vi "FCI_Lip_Outer_Width.vi"(0 "Image":T10(plugin-control), 1 "Calibrated Image":T10, 2 "Blob Center":cluster{"Center X":dbl, "Center Y":dbl}, 3 "Line Options ROI Ref":T8={"Number of Lines"=1, "Type"=enum."First Edge Rake", "Min. Score"=10.0, "Max. Score"=1000.0, "Orientation"=5.0, "Angle Range"=70.0, "Angle Tolerance"=1.0, "Step Size"=3, "Min. SNR (db)"=0.0, "Min. Points (%)"=25.0, "Hough Iterations"=5} {"Min. Points (%)" min=0.0 max=100.0; "Min. SNR (db)" min=0.0; "Max. Score" min=0.0 max=1024.0; "Min. Score" min=0.0 max=1024.0 step=1.0}, 4 "Edge Options ROI Ref":T6={"Edge Polarity"=0, "Kernel Size"=3, "Width"=3, "Minimum Edge Strength"=50.0, "Interpolation Type"=enum."Zero Order", "Data Processing Method"=enum."Average"} {"Edge Polarity" items=["All Edges", "Rising Edges", "Falling Edges"]; "Minimum Edge Strength" format="%.2f"; "Width" step=2; "Kernel Size" step=2}, 5 "error in (no error)":errorcluster, 6 "Search Direction ROI Ref":u32=3, 7 "Edge Options ROI 1":T6={"Edge Polarity"=0, "Kernel Size"=3, "Width"=3, "Minimum Edge Strength"=50.0, "Interpolation Type"=enum."Bilinear Fixed", "Data Processing Method"=enum."Average"} {"Edge Polarity" items=["All Edges", "Rising Edges", "Falling Edges"]; "Minimum Edge Strength" format="%.2f"; "Width" step=2; "Kernel Size" step=2}, 8 "Reference ROI":T11 {"Contours"."Type" items=["No Selection", "Point", "Line", "Rectangle", "Oval", "Polygon", "Freehand Region", "Annulus", "Unused2", "Unused3", "Broken Line", "Freehand Line", "Rotated Rectangle"]}, 9 "Measurement ROI":T11 {"Contours"."Type" items=["No Selection", "Point", "Line", "Rectangle", "Oval", "Polygon", "Freehand Region", "Annulus", "Unused2", "Unused3", "Broken Line", "Freehand Line", "Rotated Rectangle"]}, 10 "Search Direction ROI 1":u16(ring)=2 items=["Left To Right", "Right To Left", "Top To Bottom", "Bottom To Top"]) -> (13 "Overlay Arrow Lines":T1, 14 "Lip Outer Width Real World":sgl, 15 "Perpendicular Lines Lip Outer":T4(array[cluster])=[{{"X"=55.0, "Y"=48.0}, {"X"=263.0, "Y"=104.0}}, {{"X"=53.0, "Y"=53.0}, {"X"=262.0, "Y"=109.0}}, {{"X"=52.0, "Y"=58.0}, {"X"=261.0, "Y"=113.0}}, {{"X"=51.0, "Y"=62.0}, {"X"=259.0, "Y"=118.0}}, {{"X"=49.0, "Y"=67.0}, {"X"=258.0, "Y"=123.0}}, {{"X"=48.0, "Y"=72.0}, {"X"=257.0, "Y"=128.0}}, {{"X"=47.0, "Y"=77.0}, {"X"=255.0, "Y"=133.0}}, {{"X"=46.0, "Y"=82.0}, {"X"=254.0, "Y"=138.0}}, {{"X"=44.0, "Y"=87.0}, {"X"=253.0, "Y"=142.0}}, {{"X"=43.0, "Y"=91.0}, {"X"=252.0, "Y"=147.0}}, {{"X"=42.0, "Y"=96.0}, {"X"=250.0, "Y"=152.0}}] {"?"."Y" format="%.2f"; "?"."X" format="%.2f"; "?"."Y" format="%.2f"; "?"."X" format="%.2f"}, 19 "error IO":errorcluster)   [LabVIEW 2019, in "Algorithm.lvclass"]
uses:
  FrameworkOverrides/Algorithm.lvclass
  <vilib>/vision/NI_Vision_Development_Module.lvlib
  <vilib>/vision/Measure.llb/Edge Polarity.ctl
  <vilib>/vision/Measure.llb/Edge Options.ctl
  <vilib>/vision/Image Controls.llb/IMAQ Image.ctl
  <vilib>/vision/Measure.llb/Straight Edge Process.ctl
  <vilib>/vision/Measure.llb/Straight Edge Options.ctl
panel:
  out "Second Overlay Line":T2
  out "First Overlay Line":T3
  out "Rectangle 2":T5 {"Rotation" min=-90.0 max=90.0 step=1.0 format="%.2f"; "Left" scale=0.0..1024.0; "Right" scale=0.0..1024.0}
  out "Rectangle":T5 {"Rotation" min=-90.0 max=90.0 step=1.0 format="%.2f"; "Left" scale=0.0..1024.0; "Right" scale=0.0..1024.0}
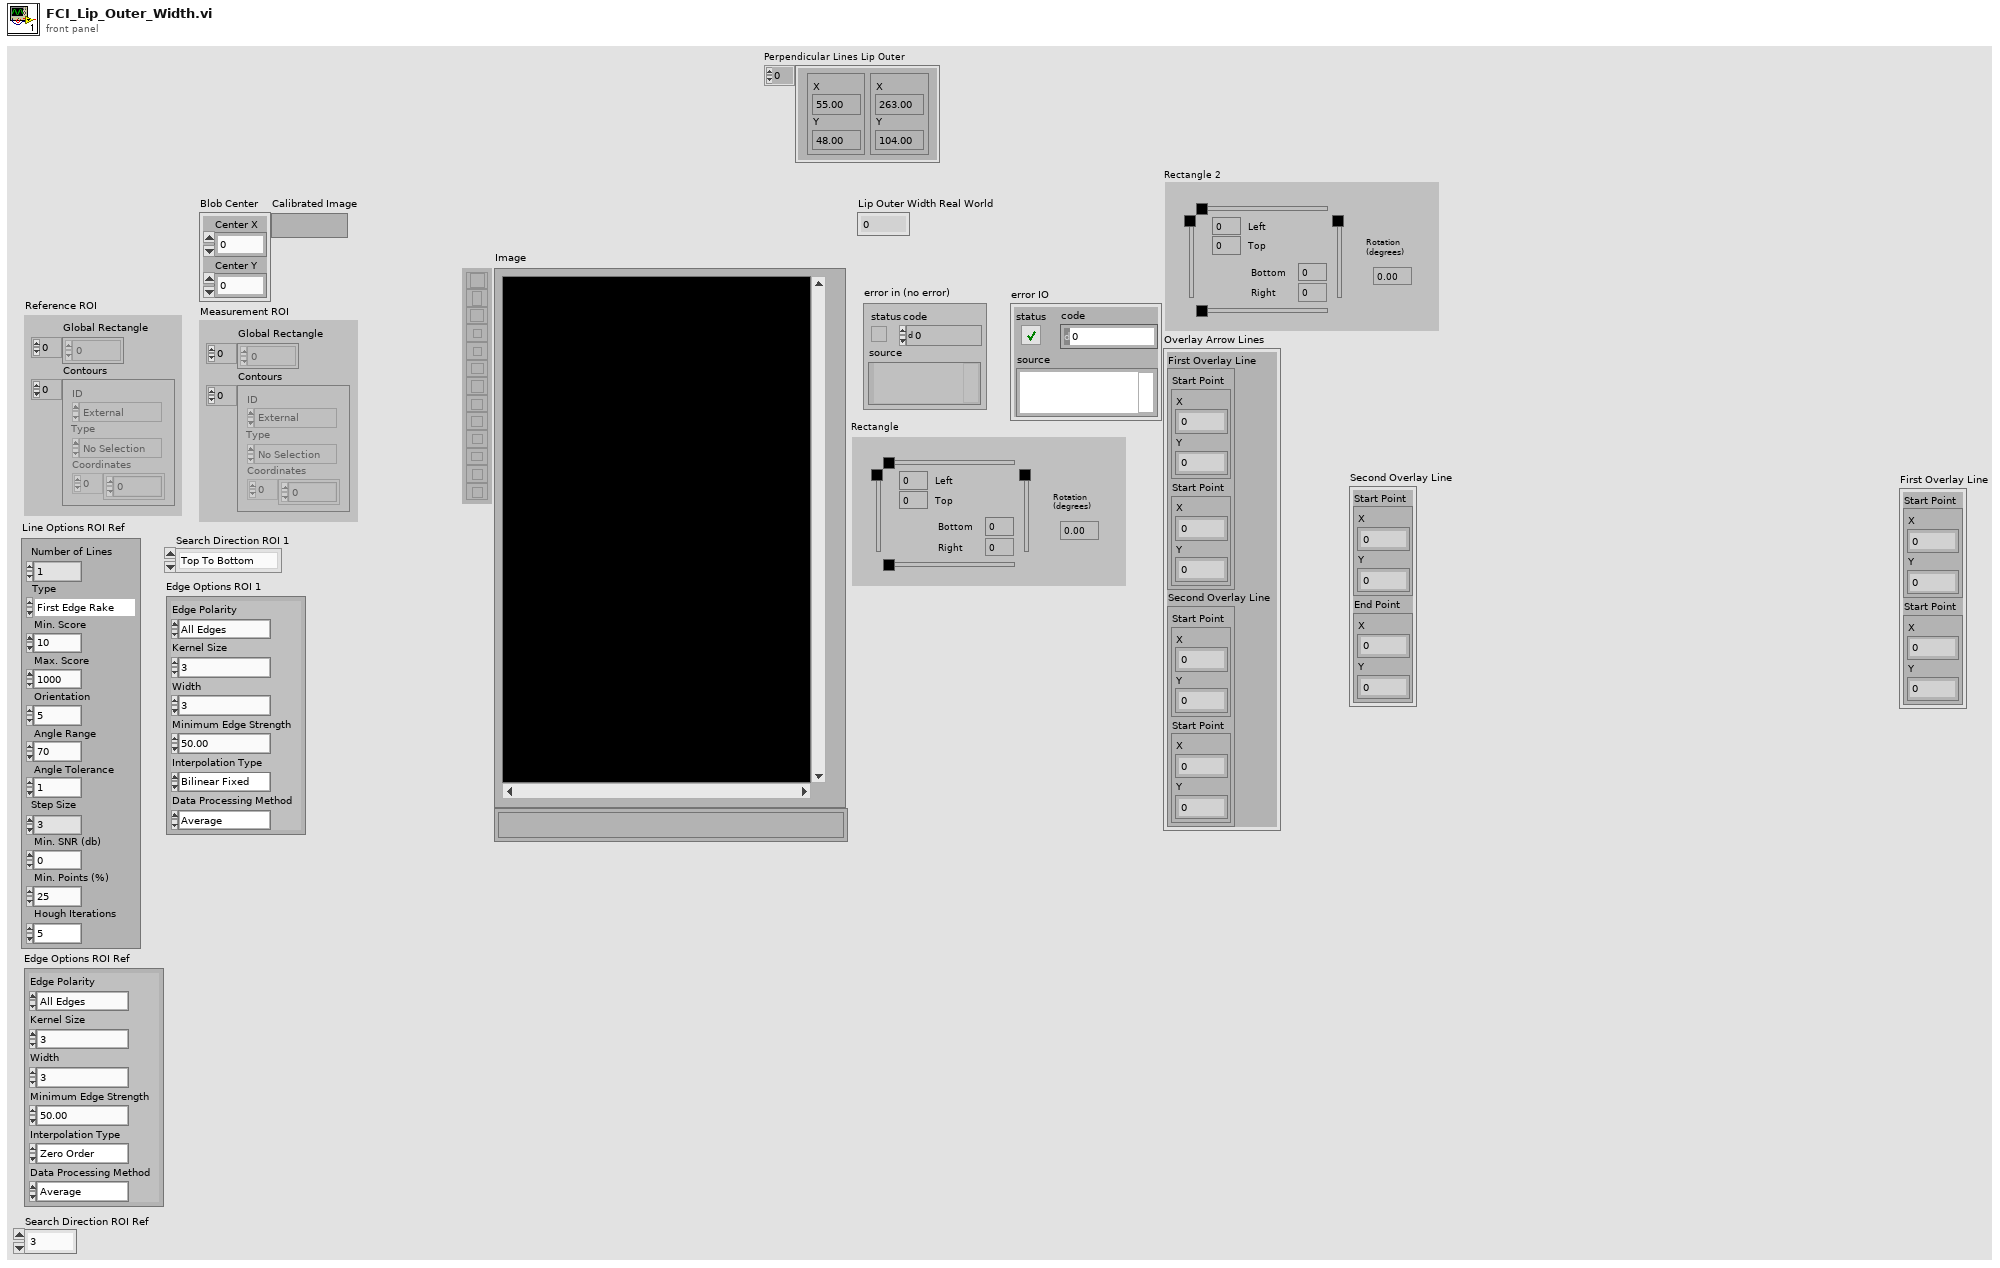
[diagram p1: front panel]
types:
  T1 = cluster{"First Overlay Line ":cluster{"Start Point":cluster{"X":sgl, "Y":sgl}, "Start Point":cluster{"X":sgl, "Y":sgl}}, "Second Overlay Line ":cluster{"Start Point":cluster{"X":sgl, "Y":sgl}, "Start Point":cluster{"X":sgl, "Y":sgl}}}
  T2 = cluster{"Start Point":cluster{"X":sgl, "Y":sgl}, "End Point":cluster{"X":sgl, "Y":sgl}}
  T3 = cluster{"Start Point":cluster{"X":sgl, "Y":sgl}, "Start Point":cluster{"X":sgl, "Y":sgl}}
  T4 = cluster{cluster{"X":sgl, "Y":sgl}, cluster{"X":sgl, "Y":sgl}}[]
  T5 = typedef "IMAQ Rectangle" = cluster{"Left":i32, "Top":i32, "Right":i32, "Bottom":i32, "Rotation":dbl}
  T6 = typedef "Edge Options.ctl" = cluster{"Edge Polarity":T7, "Kernel Size":u32, "Width":u32, "Minimum Edge Strength":sgl, "Interpolation Type":enum32{"Zero Order", "Bilinear", "Quadratic", "Cubic", "Bilinear Fixed"}, "Data Processing Method":enum32{"Average", "Median"}}
  T7 = typedef "Edge Polarity.ctl" = u32
  T8 = typedef "Straight Edge Options.ctl" = cluster{"Number of Lines":i32, "Type":T9, "Min. Score":dbl, "Max. Score":dbl, "Orientation":dbl, "Angle Range":dbl, "Angle Tolerance":dbl, "Step Size":u32, "Min. SNR (db)":dbl, "Min. Points (%)":dbl, "Hough Iterations":i32}
  T9 = typedef "Straight Edge Process.ctl" = enum32{"First Edge Rake", "Best Edge Rake", "Hough Edge Rake", "First Edge Projection", "Best Edge Projection"}
  T10 = typedef "IMAQ Image.ctl" = refnum<image>
  T11 = typedef "ROI Descriptor" = cluster{"Global Rectangle":i32[], "Contours":cluster{"ID":enum32{"External", "Internal"}, "Type":u32, "Coordinates":i32[]}[]}
  T12 = cluster{"Left":dbl, "Top":dbl, "Right":dbl, "Bottom":dbl, "Angle":dbl}
  T13 = cluster{"Search Direction":u32, "Edge Options":T6, "Show Search Area":bool, "Show Search Lines":bool, "Show Edges Found":bool, "Show Result":bool, "Search Area Color":u32, "Search Lines Color":u32, "Edge Locations Color":u32, "Result Color":u32, "Overlay Group Name":string}
  T14 = cluster{"Point1 (Pixels)":cluster{"X":sgl, "Y":sgl}, "Point2 (Pixels)":cluster{"X":sgl, "Y":sgl}, "Point1 (Real-World)":cluster{"X":sgl, "Y":sgl}, "Point2 (Real-World)":cluster{"X":sgl, "Y":sgl}, "Angle (Pixel)":dbl, "Angle (Real-World)":dbl, "Score":dbl, "Straightness":dbl, "Average SNR (db)":dbl, "Calibration Valid":bool}[]
  T15 = cluster{"Point1 (Pixels)":cluster{"X":sgl, "Y":sgl}, "Point2 (Pixels)":cluster{"X":sgl, "Y":sgl}, "Point1 (Real-World)":cluster{"X":sgl, "Y":sgl}, "Point2 (Real-World)":cluster{"X":sgl, "Y":sgl}, "Angle (Pixel)":dbl, "Angle (Real-World)":dbl, "Score":dbl, "Straightness":dbl, "Average SNR (db)":dbl, "Calibration Valid":bool}
  T16 = typedef "Search Line.ctl" = cluster{"Start Point":cluster{"X":sgl, "Y":sgl}, "End Point":cluster{"X":sgl, "Y":sgl}, "Edge Info":T17[], "Edge Map":dbl[], "Calibration Valid":bool}
  T17 = typedef "Edge New.ctl" = cluster{"Location (Pixel)":cluster{"X":sgl, "Y":sgl}, "Location (Real-World)":cluster{"X":sgl, "Y":sgl}, "Distance (Pixel)":dbl, "Distance (Real-World)":dbl, "Strength":dbl, "Noise":dbl, "Rising?":bool}
  T18 = cluster{"Start Point":cluster{"X":sgl, "Y":sgl}, cluster{"X":sgl, "Y":sgl}}
  T19 = cluster{cluster{"X":sgl, "Y":sgl}, "End Point":cluster{"X":sgl, "Y":sgl}}
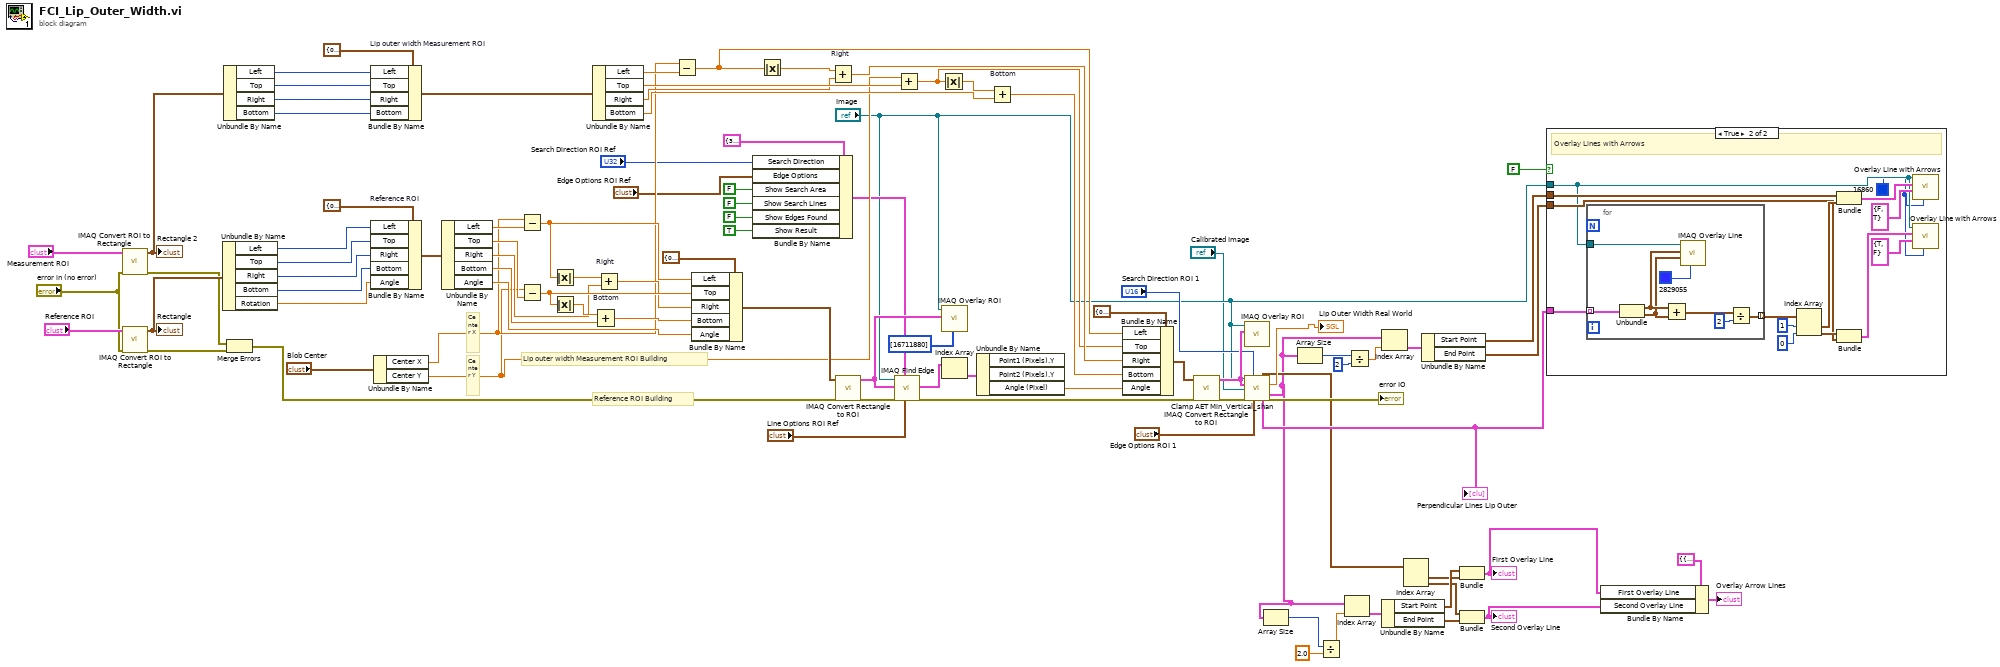
[diagram p0: block diagram]
diagram:
  # "Lip outer width Measurement ROI Building"
  # "Reference ROI Building"
  # "Center Y"
  # "Center X"
  n1 = call "IMAQ Convert ROI to Rectangle"("error in (no error)"="error in (no error)", "ROI Descriptor"="Measurement ROI") -> ("error out"=w39:errorcluster, "Rectangle"=w53:T5)  [unwired: 7 in]
  "Rectangle 2" <- w53
  n2 = call "IMAQ Convert ROI to Rectangle"("error in (no error)"="error in (no error)", "ROI Descriptor"="Reference ROI") -> ("error out"=w38:errorcluster, "Rectangle"=w46:T5)  [unwired: 7 in]
  "Rectangle" <- w46
  n3 = Unbundle By Name(w46) -> ("Left"=w45:i32, "Top"=w44:i32, "Right"=w43:i32, "Bottom"=w42:i32, "Rotation"=w41:dbl)
  n4 = Unbundle By Name(w53) -> ("Left"=w51:i32, "Top"=w50:i32, "Right"=w49:i32, "Bottom"=w48:i32)
  n5 = Merge Errors(w39, w38) -> (w37:errorcluster)
  n6 = Bundle By Name "Lip outer width Measurement ROI"(cluster=T12 {"Left"=0.0, "Top"=0.0, "Right"=0.0, "Bottom"=0.0, "Angle"=0.0} ("input cluster"), "Left"=w51, "Top"=w50, "Right"=w49, "Bottom"=w48) -> (w62:T12)
  n7 = Bundle By Name "Reference ROI"(cluster=T12 {"Left"=0.0, "Top"=0.0, "Right"=0.0, "Bottom"=0.0, "Angle"=0.0} ("input cluster"), "Left"=w45, "Top"=w44, "Right"=w43, "Bottom"=w42, "Angle"=w41) -> (w61:T12)
  n8 = Unbundle By Name("Blob Center") -> ("Center X"=w55:dbl, "Center Y"=w54:dbl)
  n9 = Unbundle By Name(w61) -> ("Left"=w88:dbl, "Top"=w87:dbl, "Right"=w86:dbl, "Bottom"=w85:dbl, "Angle"=w84:dbl)
  n10 = Subtract(x=w55, y=w88) -> (x-y=w92:dbl)
  n11 = Subtract(x=w54, y=w87) -> (x-y=w91:dbl)
  n12 = Absolute Value(x=w92) -> (abs(x)=w95:dbl)
  n13 = Absolute Value(x=w91) -> (abs(x)=w94:dbl)
  n14 = Unbundle By Name(w62) -> ("Left"=w71:dbl, "Top"=w70:dbl, "Right"=w69:dbl, "Bottom"=w68:dbl)
  n15 = Add "Bottom"(x=w94, y=w85) -> (x+y=w89:dbl)
  n16 = Add "Right"(x=w95, y=w86) -> (x+y=w90:dbl)
  n17 = Subtract(x=w55, y=w71) -> (x-y=w74:dbl)
  n18 = Bundle By Name(cluster=T12 {"Left"=0.0, "Top"=0.0, "Right"=0.0, "Bottom"=0.0, "Angle"=0.0} ("input cluster"), "Left"=w92, "Top"=w91, "Right"=w90, "Bottom"=w89, "Angle"=w84) -> (w79:T12)
  n19 = Bundle By Name(cluster=T13 {"Search Direction"=3, "Edge Options"={"Edge Polarity"=0, "Kernel Size"=3, "Width"=3, "Minimum Edge Strength"=50.0, "Interpolation Type"=enum."Zero Order", "Data Processing Method"=enum."Average"}, "Show Search Area"=FALSE, "Show Search Lines"=FALSE, "Show Edges Found"=FALSE, "Show Result"=TRUE, "Search Area Color"=65280, "Search Lines Color"=255, "Edge Locations Color"=16776960, "Result Color"=16711680, "Overlay Group Name"=""} ("Options"), "Search Direction"="Search Direction ROI Ref", "Edge Options"="Edge Options ROI Ref", "Show Search Area"=FALSE, "Show Search Lines"=FALSE, "Show Edges Found"=FALSE, "Show Result"=TRUE) -> (w32:T13)
  n20 = Absolute Value(x=w74) -> (abs(x)=w76:dbl)
  n21 = Add "Right"(x=w76, y=w69) -> (x+y=w73:dbl)
  n22 = call "IMAQ Convert Rectangle to ROI"("error in (no error)"=w37, "Rectangle"=w79) -> ("error out"=w83:errorcluster, "ROI Descriptor"=w77:T11)  [unwired: 7 in]
  n23 = call "IMAQ Find Edge"("Line Fit Options"="Line Options ROI Ref", "Options"=w32, "error in (no error)"=w83, "ROI Descriptor"=w77, "Image"="Image") -> ("error out"=w36:errorcluster, "Straight Edges"=w81:T14)  [unwired: 3 in, 2 out]
  n24 = Add(x=w54, y=w70) -> (x+y=w66:dbl)
  n25 = Absolute Value(x=w66) -> (abs(x)=w67:dbl)
  n26 = call "IMAQ Overlay ROI"("Colors (Green)"=u32[] [16711880], "ROI Descriptor"=w77, "Image"="Image") -> ()  [unwired: 7 in, 2 out]
  n27 = Index Array(array=w81) -> (element=w80:T15)  [unwired: 1 in]
  n28 = Unbundle By Name(w80) -> ("Angle (Pixel)"=w64:dbl)  [unwired: 2 out]
  n29 = Add "Bottom"(x=w67, y=w68) -> (x+y=w72:dbl)
  n30 = Bundle By Name(cluster=T12 {"Left"=0.0, "Top"=0.0, "Right"=0.0, "Bottom"=0.0, "Angle"=0.0} ("input cluster"), "Left"=w74, "Top"=w66, "Right"=w73, "Bottom"=w72, "Angle"=w64) -> (w65:T12)
  n31 = call "IMAQ Convert Rectangle to ROI"("error in (no error)"=w36, "Rectangle"=w65) -> ("error out"=w60:errorcluster, "ROI Descriptor"=w59:T11)  [unwired: 7 in]
  n32 = call "IMAQ Overlay ROI"("ROI Descriptor"=w59, "Image"="Image") -> ()  [unwired: 8 in, 2 out]
  n33 = call "Clamp AET Min_Vertical_shan.vi"("Image"="Image", "Scanning axis"="Search Direction ROI 1", "ROI Descriptor"=w59, "Calibrated Image"="Calibrated Image", "error in (no error)"=w60, "Edge Options"="Edge Options ROI 1") -> ("Edge Coordinates"=w3:cluster{"X":sgl, "Y":sgl}[], "Distance"=→"Lip Outer Width Real World":sgl, "Search Lines"=w2:T16[], "Perpendicular Lines"=w22:T4, "error out"=→"error IO":errorcluster)  [unwired: 3 in, 2 out]
  "Perpendicular Lines Lip Outer" <- w22
  n34 = Array Size(array=w2) -> (size(s)=w5:i32)
  n35 = Array Size(array=w2) -> (size(s)=w25:i32)
  n36 = Divide(x=w5, y=2.0) -> (x/y=w4:dbl)
  n37 = Index Array(array=w2, index=w4) -> (element=w14:T16)
  n38 = Divide(x=w25, y=2) -> (x/y=w23:dbl)
  n39 = Unbundle By Name(w14) -> ("Start Point"=w13:cluster{"X":sgl, "Y":sgl}, "End Point"=w10:cluster{"X":sgl, "Y":sgl})
  n40 = Index Array(array=w2, index=w23) -> (element=w26:T16)
  n41 = Index Array(array=w3) -> (element #1=w12:cluster{"X":sgl, "Y":sgl}, element #2=w11:cluster{"X":sgl, "Y":sgl})  [unwired: 2 in]
  n42 = Unbundle By Name(w26) -> ("Start Point"=w21:cluster{"X":sgl, "Y":sgl}, "End Point"=w20:cluster{"X":sgl, "Y":sgl})
  n43 = Bundle("Start Point"=w13, w12) -> (w8:T18)  [unwired: 1 in]
  "First Overlay Line" <- w8
  n44 = Bundle(w11, "End Point"=w10) -> (w7:T19)  [unwired: 1 in]
  "Second Overlay Line" <- w7
  n45 = case shown="True" FALSE {
    tunnel: w22 -> [_ w109]
    tunnel: w21 -> [_ w107]
    tunnel: w20 -> [_ w102]
    tunnel: "Image" -> [_ w97]
    frame False {
    }
    frame True {
      w96 = u32 16860 ("Color")
      # "Overlay Lines with Arrows"
      n46 = for {
        tunnel: w109 -> [w117] mode=indexing
        tunnel: w97 -> [w116]
        tunnel: [w110] -> w108 mode=indexing
        n47 = Unbundle(w117) -> (w114:cluster{"X":sgl, "Y":sgl}, w113:cluster{"X":sgl, "Y":sgl})
        n48 = Add(x=w114, y=w113) -> (x+y=w112:cluster{"X":sgl, "Y":sgl})
        n49 = call "IMAQ Overlay Line"("Color"=u32 2829055, "End Point"=w113, "Start Point"=w114, "Image"=w116) -> ()  [unwired: 6 in, 2 out]
        n50 = Divide(x=w112, y=2) -> (x/y=w110:cluster{"X":sgl, "Y":sgl})
      }
      n51 = Index Array(array=w108, index #1=1 ("index"), index #2=0 ("index")) -> (element #1=w105:cluster{"X":sgl, "Y":sgl}, element #2=w103:cluster{"X":sgl, "Y":sgl})
      n52 = Bundle("Start Point"=w107, w105) -> (w101:T18)  [unwired: 1 in]
      n53 = Bundle(w103, "End Point"=w102) -> (w99:T19)  [unwired: 1 in]
      n54 = call <vilib>:"Overlay Line with Arrows.vi"("Color"=w96, "Arrows"=cluster{"Start point":bool, "End point":bool} {"Start point"=FALSE, "End point"=TRUE}, "Line Coordinates"=w101, "Image In"=w97) -> ()  [unwired: 6 in, 2 out]
      n55 = call <vilib>:"Overlay Line with Arrows.vi"("Color"=w96, "Arrows"=cluster{"Start point":bool, "End point":bool} {"Start point"=TRUE, "End point"=FALSE}, "Line Coordinates"=w99, "Image In"=w97) -> ()  [unwired: 6 in, 2 out]
    }
  }
  n56 = Bundle By Name(cluster=T1 {"First Overlay Line "={"Start Point"={"X"=0.0, "Y"=0.0}, "Start Point"={"X"=0.0, "Y"=0.0}}, "Second Overlay Line "={"Start Point"={"X"=0.0, "Y"=0.0}, "Start Point"={"X"=0.0, "Y"=0.0}}}, "First Overlay Line"=w8, "Second Overlay Line"=w7) -> (→"Overlay Arrow Lines":T1)
